vi "Create measurement file.vi"(4 "error in":errorcluster, 5 "input main cluster":T1) -> (0 "error out":errorcluster, 1 "output main cluster":T1, 3 "refnum out":refnum<file>)   [LabVIEW 2010]
uses:
  Main_cluster.ctl
  <vilib>/vision/Image Controls.llb/IMAQ Image.ctl
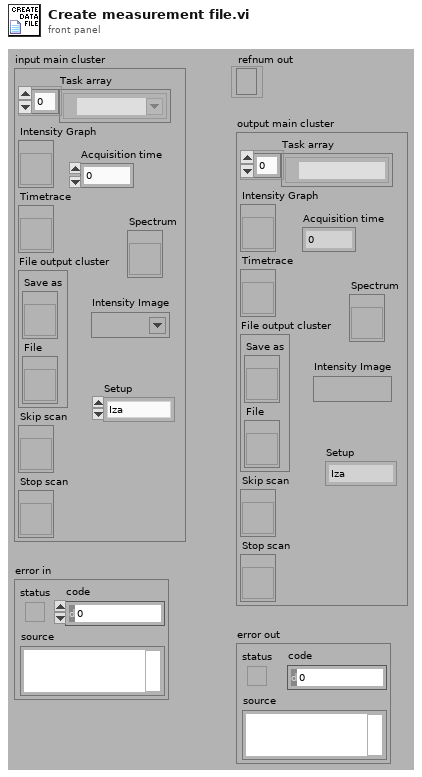
[diagram p1: front panel]
types:
  T1 = typedef "Main_cluster.ctl" = cluster{"Task array":refnum<k21>[], "Intensity Graph":refnum<vi>, "Timetrace":refnum<vi>, "File output cluster":cluster{"Save as":refnum<vi>, "File":refnum<vi>}, "Skip scan":refnum<vi>, "Stop scan":refnum<vi>, "Acquisition time":dbl, "Setup":enum16{"Iza", "Lukasz"}, "Spectrum":refnum<vi>, "Intensity Image":T2}
  T2 = typedef "IMAQ Image.ctl" = refnum<image>
  T3 = enum16{"open", "replace", "create", "open or create", "replace or create", "replace or create with confirmation"}
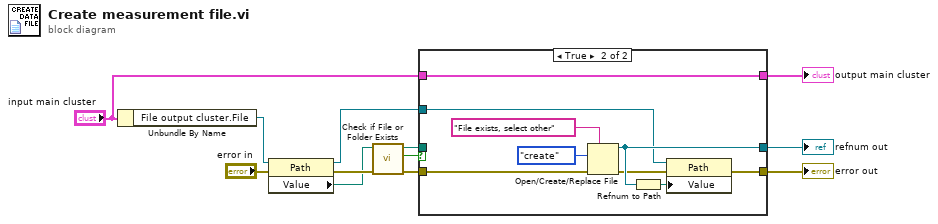
[diagram p0: block diagram]
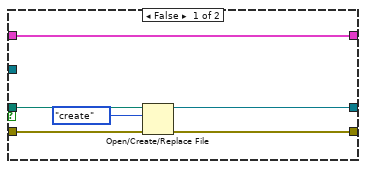
[diagram p2: hidden frame]
diagram:
  n1 = Unbundle By Name("input main cluster") -> ("File output cluster.File"=w4:refnum<vi>)
  n2 = property class="Path"(reference=w4, error in="error in") -> (reference out=w12:refnum<vi>, error out=w5:errorcluster, "Value"=w3:path)
  n3 = call <vilib>:"Check if File or Folder Exists.vi"("error in (no error)"=w5, "path"=w3) -> ("error out"=w8:errorcluster, "file or folder exists?"=w2:bool, "dup path"=w7:path)  [unwired: 7 in]
  n4 = case shown="True" w2 {
    tunnel: w7 -> [w17 _]
    tunnel: w8 -> [w16 w26]
    tunnel: [w14 w19] -> w9
    tunnel: [w15 w23] -> w1
    tunnel: [w13 w24] -> w10
    tunnel: "input main cluster" -> [w13 w24]
    tunnel: w12 -> [_ w21]
    frame False {
      n5 = Open/Create/Replace File(file path (use dialog)=w17, error in=w16, operation (0:open)=T3."create") -> (refnum out=w15:refnum<file>, error out=w14:errorcluster)  [unwired: 3 in, 1 out]
    }
    frame True {
      n6 = Open/Create/Replace File(error in=w26, prompt="File exists, select other", operation (0:open)=T3."create") -> (refnum out=w23:refnum<file>, error out=w20:errorcluster)  [unwired: 3 in, 1 out]
      n7 = Refnum to Path(1:w23) -> (0:w22:path)
      n8 = property class="Path"(reference=w21, error in=w20, "Value"=w22) -> (error out=w19:errorcluster)  [unwired: 1 out]
    }
  }
  "output main cluster" <- w10
  "error out" <- w9
  "refnum out" <- w1
